vi "RC control.vi"(8 "error in (no error)":errorcluster, 10 "position":i32, 11 "KNR in":T1) -> (0 "error out":errorcluster, 3 "KNR out":T1)   [LabVIEW 2013]
uses:
  <userlib>/KNR OS 3.0 LabVIEW Toolkit/Type Definition/KNR3 Reference.ctl
  <userlib>/_FPGA Interface Advanced Tools/FPGA Interface Base/FPGA Interface Base.lvclass
  <userlib>/KNR OS 3.0 LabVIEW Toolkit/Type Definition/Resource.ctl
  <userlib>/KNR OS 3.0 LabVIEW Toolkit/Type Definition/RC Servo Port.ctl
panel:
  out "output array":u16[](array[numeric])
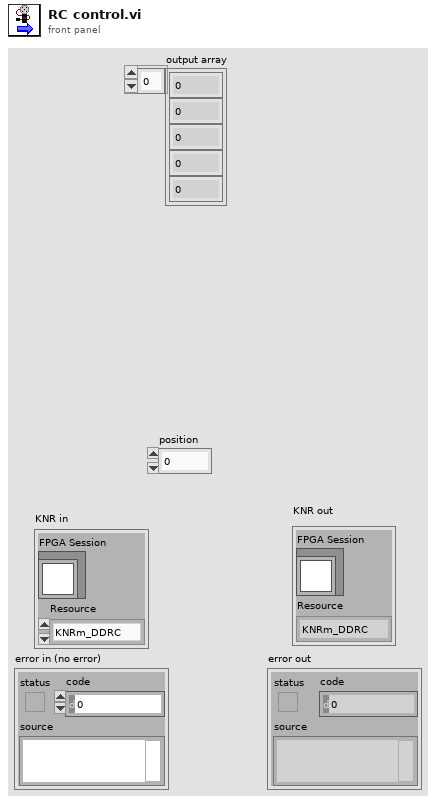
[diagram p1: front panel]
types:
  T1 = typedef "KNR3 Reference.ctl" = cluster{"FPGA Session":refnum<class "FPGA Interface Base.lvclass">, "Resource":T2}
  T2 = typedef "Resource.ctl" = enum16{"KNRm_DDRC", "KNRm_DDDD", "KNRm_DDDR", "KNRm_DDDC", "KNR"}
  T3 = typedef "RC Servo Port.ctl" = u16
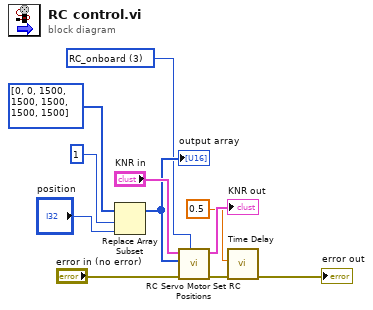
[diagram p0: block diagram]
diagram:
  w6 = T3 3 items=["RC_onboard"=3, "RC_box"=9] ("Port (RC_onboard)")
  n1 = Replace Array Subset(array=u16[] [0, 0, 1500, 1500, 1500, 1500, 1500] ("RC Pulse Width (1500 uS)"), new element="position", index=1) -> (w7:u16[])
  "output array" <- w7
  n2 = call <userlib>:"RC Servo Motor Set RC Positions.vi"("Port (RC_onboard)"=w6, "error in (no error)"="error in (no error)", "RC Pulse Width (1500 uS)"=w7, "KNR in"="KNR in") -> ("error out"=w4:errorcluster, "KNR out"=→"KNR out":T1)  [unwired: 6 in]
  n3 = call "Time Delay"("error in (no error)"=w4, "Delay Time (s)"=0.5) -> ("error out"=→"error out":errorcluster)  [unwired: 9 in]
